vi "S4GUI_002.vi"(7 "Tab ObsEng":enum32{"Obs", "CCD modes", "Eng"}(tab)) -> ()   [LabVIEW 2018] (continued)
            n3950 = call-dynamic "Read AcquisitionA.vi"("error in (no error)"=w9244, "S4ACS_GUI in"=w9246) -> ("error out"=w9249:errorcluster, "Acquisition.lvclass"=w9248:refnum<class "Acquisition.lvclass">, "S4ACS_GUI out"=w9245:refnum<class "S4GUI.lvclass">)  [unwired: 7 in]
            n3951 = call-dynamic "Read Channel.vi"("error in (no error)"=w9249, "Acquisition in"=w9248) -> ("error out"=w9251:errorcluster, "Channel.lvclass"=w9250:refnum<class "Channel.lvclass">, "Acquisition out"=w9259:refnum<class "Acquisition.lvclass">)  [unwired: 7 in]
            n3952 = call-dynamic "Read State Machine.vi"("error in (no error)"=w9251, "Device in"=w9250) -> ("error out"=w9253:errorcluster, "State Machine.lvclass"=w9252:refnum<class "State Machine.lvclass">, "Device out"=w9255:refnum<class "Channel.lvclass">)  [unwired: 7 in]
            n3953 = call "Next State.vi"("error in (no error)"=w9253, "New_State"=u32 80, "State Machine in"=w9252) -> ("error out"=w9256:errorcluster, "State Machine out"=w9254:refnum<class "State Machine.lvclass">)  [unwired: 7 in]
            n3954 = call-dynamic "Write State Machine.vi"("error in (no error)"=w9256, "State Machine.lvclass"=w9254, "Device in"=w9255) -> ("error out"=w9260:errorcluster, "Device out"=w9261:refnum<class "Channel.lvclass">)  [unwired: 7 in]
            n3955 = call-dynamic "Write Channel.vi"("error in (no error)"=w9260, "Channel.lvclass"=w9261, "Acquisition in"=w9259) -> ("error out"=w9258:errorcluster, "Acquisition out"=w9257:refnum<class "Acquisition.lvclass">)  [unwired: 7 in]
            n3956 = call-dynamic "Write AcquisitionA.vi"("error in (no error)"=w9258, "Acquisition.lvclass"=w9257, "S4ACS_GUI in"=w9245) -> ("error out"=w9230:errorcluster, "S4ACS_GUI out"=w9229:refnum<class "S4GUI.lvclass">)  [unwired: 7 in]
            n3957 = call "Read AcquisitionB.vi"("error in (no error)"=w9230, "S4ACS_GUI in"=w9229) -> ("error out"=w9223:errorcluster, "Acquisition.lvclass"=w9227:refnum<class "Acquisition.lvclass">, "S4ACS_GUI out"=w9228:refnum<class "S4GUI.lvclass">)  [unwired: 7 in]
            n3958 = call-dynamic "Read Channel.vi"("error in (no error)"=w9223, "Acquisition in"=w9227) -> ("error out"=w9238:errorcluster, "Channel.lvclass"=w9239:refnum<class "Channel.lvclass">, "Acquisition out"=w9225:refnum<class "Acquisition.lvclass">)  [unwired: 7 in]
            n3959 = call-dynamic "Read State Machine.vi"("error in (no error)"=w9238, "Device in"=w9239) -> ("error out"=w9236:errorcluster, "State Machine.lvclass"=w9237:refnum<class "State Machine.lvclass">, "Device out"=w9234:refnum<class "Channel.lvclass">)  [unwired: 7 in]
            n3960 = call "Next State.vi"("error in (no error)"=w9236, "New_State"=u32 80, "State Machine in"=w9237) -> ("error out"=w9233:errorcluster, "State Machine out"=w9235:refnum<class "State Machine.lvclass">)  [unwired: 7 in]
            n3961 = call-dynamic "Write State Machine.vi"("error in (no error)"=w9233, "State Machine.lvclass"=w9235, "Device in"=w9234) -> ("error out"=w9232:errorcluster, "Device out"=w9231:refnum<class "Channel.lvclass">)  [unwired: 7 in]
            n3962 = call-dynamic "Write Channel.vi"("error in (no error)"=w9232, "Channel.lvclass"=w9231, "Acquisition in"=w9225) -> ("error out"=w9224:errorcluster, "Acquisition out"=w9226:refnum<class "Acquisition.lvclass">)  [unwired: 7 in]
            n3963 = call "Write AcquisitionB.vi"("error in (no error)"=w9224, "Acquisition.lvclass"=w9226, "S4ACS_GUI in"=w9228) -> ("error out"=w9190:errorcluster, "S4ACS_GUI out"=w9189:refnum<class "S4GUI.lvclass">)  [unwired: 7 in]
            n3964 = call-dynamic "Read AcquisitionC.vi"("error in (no error)"=w9190, "S4ACS_GUI in"=w9189) -> ("error out"=w9207:errorcluster, "Acquisition.lvclass"=w9211:refnum<class "Acquisition.lvclass">, "S4ACS_GUI out"=w9212:refnum<class "S4GUI.lvclass">)  [unwired: 7 in]
            n3965 = call-dynamic "Read Channel.vi"("error in (no error)"=w9207, "Acquisition in"=w9211) -> ("error out"=w9220:errorcluster, "Channel.lvclass"=w9221:refnum<class "Channel.lvclass">, "Acquisition out"=w9209:refnum<class "Acquisition.lvclass">)  [unwired: 7 in]
            n3966 = call-dynamic "Read State Machine.vi"("error in (no error)"=w9220, "Device in"=w9221) -> ("error out"=w9218:errorcluster, "State Machine.lvclass"=w9219:refnum<class "State Machine.lvclass">, "Device out"=w9216:refnum<class "Channel.lvclass">)  [unwired: 7 in]
            n3967 = call "Next State.vi"("error in (no error)"=w9218, "New_State"=u32 80, "State Machine in"=w9219) -> ("error out"=w9215:errorcluster, "State Machine out"=w9217:refnum<class "State Machine.lvclass">)  [unwired: 7 in]
            n3968 = call-dynamic "Write State Machine.vi"("error in (no error)"=w9215, "State Machine.lvclass"=w9217, "Device in"=w9216) -> ("error out"=w9214:errorcluster, "Device out"=w9213:refnum<class "Channel.lvclass">)  [unwired: 7 in]
            n3969 = call-dynamic "Write Channel.vi"("error in (no error)"=w9214, "Channel.lvclass"=w9213, "Acquisition in"=w9209) -> ("error out"=w9208:errorcluster, "Acquisition out"=w9210:refnum<class "Acquisition.lvclass">)  [unwired: 7 in]
            n3970 = call-dynamic "Write AcquisitionC.vi"("error in (no error)"=w9208, "Acquisition.lvclass"=w9210, "S4ACS_GUI in"=w9212) -> ("error out"=w9188:errorcluster, "S4ACS_GUI out"=w9187:refnum<class "S4GUI.lvclass">)  [unwired: 7 in]
            n3971 = call-dynamic "Read AcquisitionD.vi"("error in (no error)"=w9188, "S4ACS_GUI in"=w9187) -> ("error out"=w9191:errorcluster, "Acquisition.lvclass"=w9195:refnum<class "Acquisition.lvclass">, "S4ACS_GUI out"=w9196:refnum<class "S4GUI.lvclass">)  [unwired: 7 in]
            n3972 = call-dynamic "Read Channel.vi"("error in (no error)"=w9191, "Acquisition in"=w9195) -> ("error out"=w9204:errorcluster, "Channel.lvclass"=w9205:refnum<class "Channel.lvclass">, "Acquisition out"=w9193:refnum<class "Acquisition.lvclass">)  [unwired: 7 in]
            n3973 = call-dynamic "Read State Machine.vi"("error in (no error)"=w9204, "Device in"=w9205) -> ("error out"=w9202:errorcluster, "State Machine.lvclass"=w9203:refnum<class "State Machine.lvclass">, "Device out"=w9200:refnum<class "Channel.lvclass">)  [unwired: 7 in]
            n3974 = call "Next State.vi"("error in (no error)"=w9202, "New_State"=u32 80, "State Machine in"=w9203) -> ("error out"=w9199:errorcluster, "State Machine out"=w9201:refnum<class "State Machine.lvclass">)  [unwired: 7 in]
            n3975 = call-dynamic "Write State Machine.vi"("error in (no error)"=w9199, "State Machine.lvclass"=w9201, "Device in"=w9200) -> ("error out"=w9198:errorcluster, "Device out"=w9197:refnum<class "Channel.lvclass">)  [unwired: 7 in]
            n3976 = call-dynamic "Write Channel.vi"("error in (no error)"=w9198, "Channel.lvclass"=w9197, "Acquisition in"=w9193) -> ("error out"=w9192:errorcluster, "Acquisition out"=w9194:refnum<class "Acquisition.lvclass">)  [unwired: 7 in]
            n3977 = call-dynamic "Write AcquisitionD.vi"("error in (no error)"=w9192, "Acquisition.lvclass"=w9194, "S4ACS_GUI in"=w9196) -> ("error out"=w9185:errorcluster, "S4ACS_GUI out"=w9186:refnum<class "S4GUI.lvclass">)  [unwired: 7 in]
            n3978 = disable-structure shown="Enabled" {
              disable-tunnel: w9186 -> [w9266 w9268]
              disable-tunnel: w9185 -> [w9265 w9267]
              disable-tunnel: [w9263 w9268] -> w9242
              disable-tunnel: [w9262 w9267] -> w9241
              frame Disabled {
                n3979 = call-dynamic "Write aborted.vi"("error in (no error)"=w9265, "aborted"=TRUE ("stopped"), "S4ACS_GUI in"=w9266) -> ("error out"=w9262:errorcluster, "S4ACS_GUI out"=w9263:refnum<class "S4GUI.lvclass">)  [unwired: 7 in]
              }
              frame Enabled {
              }
            }
            n3980 = call-dynamic "Write Obs_state.vi"("error in (no error)"=w9241, "Obs_state"=u32 0, "S4ACS_GUI in"=w9242) -> ("error out"=w9159:errorcluster, "S4ACS_GUI out"=w9160:refnum<class "S4GUI.lvclass">)  [unwired: 7 in]
            n3981 = call "Read Instrument.lvclass.vi"("error in (no error)"=w9159, "S4ACS_GUI in"=w9160) -> ("error out"=w9179:errorcluster, "Instrument.lvclass"=w9181:refnum<class "Instrument.lvclass">, "S4ACS_GUI out"=w9180:refnum<class "S4GUI.lvclass">)  [unwired: 7 in]
            n3982 = call "Read WPROT.vi"("error in (no error)"=w9179, "Instrument in"=w9181) -> ("error out"=w9174:errorcluster, "Opt_Selector.lvclass"=w9177:refnum<class "Opt_Selector.lvclass">, "Instrument out"=w9182:refnum<class "Instrument.lvclass">)  [unwired: 7 in]
            n3983 = call-dynamic "Read sequencia_ant.vi"("error in (no error)"=w9174, "Opt_Selector in"=w9177) -> ("error out"=w9173:errorcluster, "sequencia_ant"=w9175:u16, "Opt_Selector out"=w9176:refnum<class "Opt_Selector.lvclass">)  [unwired: 7 in]
            n3984 = call-dynamic "Write sequencia.vi"("error in (no error)"=w9173, "sequencia"=w9175, "Opt_Selector in"=w9176) -> ("error out"=w9168:errorcluster, "Opt_Selector out"=w9169:refnum<class "Opt_Selector.lvclass">)  [unwired: 7 in]
            n3985 = call-dynamic "Read State Machine.vi"("error in (no error)"=w9168, "Device in"=w9169) -> ("error out"=w9171:errorcluster, "State Machine.lvclass"=w9166:refnum<class "State Machine.lvclass">, "Device out"=w9167:refnum<class "Opt_Selector.lvclass">)  [unwired: 7 in]
            n3986 = call "Next State.vi"("error in (no error)"=w9171, "New_State"=10, "State Machine in"=w9166) -> ("error out"=w9170:errorcluster, "State Machine out"=w9165:refnum<class "State Machine.lvclass">)  [unwired: 7 in]
            n3987 = call-dynamic "Write State Machine.vi"("error in (no error)"=w9170, "State Machine.lvclass"=w9165, "Device in"=w9167) -> ("error out"=w9164:errorcluster, "Device out"=w9163:refnum<class "Opt_Selector.lvclass">)  [unwired: 7 in]
            n3988 = call "Write WPROT.vi"("error in (no error)"=w9164, "Opt_Selector.lvclass"=w9163, "Instrument in"=w9182) -> ("error out"=w9161:errorcluster, "Instrument out"=w9162:refnum<class "Instrument.lvclass">)  [unwired: 7 in]
            n3989 = call "Write Instrument.lvclass.vi"("error in (no error)"=w9161, "Instrument.lvclass"=w9162, "S4ACS_GUI in"=w9180) -> ("error out"=w9183:errorcluster, "S4ACS_GUI out"=w9184:refnum<class "S4GUI.lvclass">)  [unwired: 7 in]
            n3990 = call-dynamic "Write ciclos.vi"("error in (no error)"=w9183, "ciclos"=u32 0, "S4ACS_GUI in"=w9184) -> ("error out"=w9157:errorcluster, "S4ACS_GUI out"=w9158:refnum<class "S4GUI.lvclass">)  [unwired: 7 in]
          }
          frame Enabled {
            w9274 = FALSE ("Wait Until Done")
            n3991 = call <vilib>:"Application Directory.vi"() -> ("Application Directory"=w9269:path)
            n3992 = Build Path(base path=w9269, name or relative path="MsgAbortSync.vi") -> (appended path=w9277:path)
            n3993 = Open VI Reference(vi path=w9277, error in (no error)=w9272) -> (vi reference=w9276:refnum<vi>, error out=w9275:errorcluster)  [unwired: 4 in]
            n3994 = invoke class="VI" method="Run VI"(reference=w9276, error in=w9275, "Wait until done"=w9274, "Auto Dispose Ref"=w9274) -> (error out=w9271:errorcluster)  [unwired: 1 in, 4 out]
          }
        }
        n3995 = property on="#Cycles Done" class="Slide (strict)"(error in=w9153, "Scale.Maximum"=w9155, "Scale.Minimum"=w9155) -> (error out=w9156:errorcluster)  [unwired: 1 in, 1 out]
      }
      event "Pause SM": Value Change {
        n3996 = event-data() -> ()  [unwired: 1 in, 6 out]
        n3997 = call-dynamic "Write User Event.vi"("error in (no error)"=w9281, "User Event"="PAUSE SM CLICKED", "S4GUI in"=w9282) -> ("error out"=w9279:errorcluster, "S4GUI out"=w9280:refnum<class "S4GUI.lvclass">)  [unwired: 7 in]
        n3998 = disable-structure shown="Enabled" {
          disable-tunnel: w9280 -> [w9296 w9306]
          disable-tunnel: w9279 -> [w9295 w9307]
          disable-tunnel: [w9286 w9306] -> w9284
          disable-tunnel: [w9285 w9305] -> w9283
          frame Disabled {
            n3999 = disable-structure shown="Enabled" {
              disable-tunnel: w9296 -> [w9300 w9303]
              disable-tunnel: w9295 -> [w9299 w9302]
              disable-tunnel: [w9298 w9303] -> w9289
              disable-tunnel: [w9297 w9302] -> w9288
              frame Disabled {
                n4000 = call-dynamic "Write paused.vi"("error in (no error)"=w9299, "paused"=TRUE ("stopped"), "S4ACS_GUI in"=w9300) -> ("error out"=w9297:errorcluster, "S4ACS_GUI out"=w9298:refnum<class "S4GUI.lvclass">)  [unwired: 7 in]
              }
              frame Enabled {
              }
            }
            n4001 = call-dynamic "Read Obs_state.vi"("error in (no error)"=w9288, "S4ACS_GUI in"=w9289) -> ("error out"=w9292:errorcluster, "Obs_state"=w9294:u32, "S4ACS_GUI out"=w9293:refnum<class "S4GUI.lvclass">)  [unwired: 7 in]
            n4002 = call-dynamic "Write Obs_prevstate.vi"("error in (no error)"=w9292, "Obs_prevstate"=w9294, "S4ACS_GUI in"=w9293) -> ("error out"=w9290:errorcluster, "S4ACS_GUI out"=w9291:refnum<class "S4GUI.lvclass">)  [unwired: 7 in]
            n4003 = call-dynamic "Write Obs_state.vi"("error in (no error)"=w9290, "Obs_state"=u32 400, "S4ACS_GUI in"=w9291) -> ("error out"=w9285:errorcluster, "S4ACS_GUI out"=w9286:refnum<class "S4GUI.lvclass">)  [unwired: 7 in]
          }
          frame Enabled {
            w9309 = FALSE ("Wait Until Done")
            n4004 = call <vilib>:"Application Directory.vi"() -> ("Application Directory"=w9304:path)
            n4005 = Build Path(base path=w9304, name or relative path="MsgPauseSync.vi") -> (appended path=w9312:path)
            n4006 = Open VI Reference(vi path=w9312, error in (no error)=w9307) -> (vi reference=w9311:refnum<vi>, error out=w9310:errorcluster)  [unwired: 4 in]
            n4007 = invoke class="VI" method="Run VI"(reference=w9311, error in=w9310, "Wait until done"=w9309, "Auto Dispose Ref"=w9309) -> (error out=w9305:errorcluster)  [unwired: 1 in, 4 out]
          }
        }
      }
      event "Abort ch1": Value Change {
        n4008 = event-data() -> ()  [unwired: 1 in, 6 out]
        n4009 = disable-structure shown="Enabled" {
          disable-tunnel: w9316 -> [w9349 w9371]
          disable-tunnel: w9315 -> [w9347 w9365]
          disable-tunnel: [w9329 w9364] -> w9314
          disable-tunnel: [w9317 w9371] -> w9313
          frame Disabled {
            # "Para movimento \nda lamina retardadora"
            # "Restaura a última sequência de lâminas"
            n4010 = call-dynamic "Read AcquisitionA.vi"("error in (no error)"=w9347, "S4ACS_GUI in"=w9349) -> ("error out"=w9352:errorcluster, "Acquisition.lvclass"=w9351:refnum<class "Acquisition.lvclass">, "S4ACS_GUI out"=w9348:refnum<class "S4GUI.lvclass">)  [unwired: 7 in]
            n4011 = call-dynamic "Read Channel.vi"("error in (no error)"=w9352, "Acquisition in"=w9351) -> ("error out"=w9354:errorcluster, "Channel.lvclass"=w9353:refnum<class "Channel.lvclass">, "Acquisition out"=w9360:refnum<class "Acquisition.lvclass">)  [unwired: 7 in]
            n4012 = call-dynamic "Read State Machine.vi"("error in (no error)"=w9354, "Device in"=w9353) -> ("error out"=w9356:errorcluster, "State Machine.lvclass"=w9355:refnum<class "State Machine.lvclass">, "Device out"=w9358:refnum<class "Channel.lvclass">)  [unwired: 7 in]
            n4013 = call "Next State.vi"("error in (no error)"=w9356, "New_State"=u32 80, "State Machine in"=w9355) -> ("error out"=w9359:errorcluster, "State Machine out"=w9357:refnum<class "State Machine.lvclass">)  [unwired: 7 in]
            n4014 = call-dynamic "Write State Machine.vi"("error in (no error)"=w9359, "State Machine.lvclass"=w9357, "Device in"=w9358) -> ("error out"=w9361:errorcluster, "Device out"=w9362:refnum<class "Channel.lvclass">)  [unwired: 7 in]
            n4015 = call-dynamic "Write Channel.vi"("error in (no error)"=w9361, "Channel.lvclass"=w9362, "Acquisition in"=w9360) -> ("error out"=w9344:errorcluster, "Acquisition out"=w9345:refnum<class "Acquisition.lvclass">)  [unwired: 7 in]
            n4016 = call-dynamic "Write Acq_state.vi"("error in (no error)"=w9344, "Acq_state"=u32 0, "Acquisition in"=w9345) -> ("error out"=w9343:errorcluster, "Acquisition out"=w9342:refnum<class "Acquisition.lvclass">)  [unwired: 7 in]
            n4017 = call-dynamic "Write AcquisitionA.vi"("error in (no error)"=w9343, "Acquisition.lvclass"=w9342, "S4ACS_GUI in"=w9348) -> ("error out"=w9330:errorcluster, "S4ACS_GUI out"=w9328:refnum<class "S4GUI.lvclass">)  [unwired: 7 in]
            n4018 = call "Read Instrument.lvclass.vi"("error in (no error)"=w9330, "S4ACS_GUI in"=w9328) -> ("error out"=w9337:errorcluster, "Instrument.lvclass"=w9340:refnum<class "Instrument.lvclass">, "S4ACS_GUI out"=w9341:refnum<class "S4GUI.lvclass">)  [unwired: 7 in]
            n4019 = call "Read WPROT.vi"("error in (no error)"=w9337, "Instrument in"=w9340) -> ("error out"=w9336:errorcluster, "Opt_Selector.lvclass"=w9338:refnum<class "Opt_Selector.lvclass">, "Instrument out"=w9339:refnum<class "Instrument.lvclass">)  [unwired: 7 in]
            n4020 = call-dynamic "Read sequencia_ant.vi"("error in (no error)"=w9336, "Opt_Selector in"=w9338) -> ("error out"=w9332:errorcluster, "sequencia_ant"=w9331:u16, "Opt_Selector out"=w9333:refnum<class "Opt_Selector.lvclass">)  [unwired: 7 in]
            n4021 = call-dynamic "Write sequencia.vi"("error in (no error)"=w9332, "sequencia"=w9331, "Opt_Selector in"=w9333) -> ("error out"=w9321:errorcluster, "Opt_Selector out"=w9322:refnum<class "Opt_Selector.lvclass">)  [unwired: 7 in]
            n4022 = call-dynamic "Read State Machine.vi"("error in (no error)"=w9321, "Device in"=w9322) -> ("error out"=w9324:errorcluster, "State Machine.lvclass"=w9327:refnum<class "State Machine.lvclass">, "Device out"=w9320:refnum<class "Opt_Selector.lvclass">)  [unwired: 7 in]
            n4023 = call "Next State.vi"("error in (no error)"=w9324, "New_State"=10, "State Machine in"=w9327) -> ("error out"=w9323:errorcluster, "State Machine out"=w9326:refnum<class "State Machine.lvclass">)  [unwired: 7 in]
            n4024 = call-dynamic "Write State Machine.vi"("error in (no error)"=w9323, "State Machine.lvclass"=w9326, "Device in"=w9320) -> ("error out"=w9318:errorcluster, "Device out"=w9319:refnum<class "Opt_Selector.lvclass">)  [unwired: 7 in]
            n4025 = call "Write WPROT.vi"("error in (no error)"=w9318, "Opt_Selector.lvclass"=w9319, "Instrument in"=w9339) -> ("error out"=w9335:errorcluster, "Instrument out"=w9334:refnum<class "Instrument.lvclass">)  [unwired: 7 in]
            n4026 = call "Write Instrument.lvclass.vi"("error in (no error)"=w9335, "Instrument.lvclass"=w9334, "S4ACS_GUI in"=w9341) -> ("error out"=w9329:errorcluster, "S4ACS_GUI out"=w9317:refnum<class "S4GUI.lvclass">)  [unwired: 7 in]
          }
          frame Enabled {
            w9367 = FALSE ("Wait Until Done")
            n4027 = call <vilib>:"Application Directory.vi"() -> ("Application Directory"=w9363:path)
            n4028 = Build Path(base path=w9363, name or relative path="MsgAbort1.vi") -> (appended path=w9370:path)
            n4029 = Open VI Reference(vi path=w9370, error in (no error)=w9365) -> (vi reference=w9369:refnum<vi>, error out=w9368:errorcluster)  [unwired: 4 in]
            n4030 = invoke class="VI" method="Run VI"(reference=w9369, error in=w9368, "Wait until done"=w9367, "Auto Dispose Ref"=w9367) -> (error out=w9364:errorcluster)  [unwired: 1 in, 4 out]
          }
        }
      }
      event "Abort ch2": Value Change {
        n4031 = event-data() -> ()  [unwired: 1 in, 6 out]
        n4032 = disable-structure shown="Enabled" {
          disable-tunnel: w9375 -> [w9408 w9424]
          disable-tunnel: w9374 -> [w9406 w9425]
          disable-tunnel: [w9388 w9423] -> w9373
          disable-tunnel: [w9376 w9424] -> w9372
          frame Disabled {
            # "Para movimento \nda lamina retardadora"
            # "Restaura a última sequência de lâminas"
            n4033 = call "Read AcquisitionB.vi"("error in (no error)"=w9406, "S4ACS_GUI in"=w9408) -> ("error out"=w9411:errorcluster, "Acquisition.lvclass"=w9410:refnum<class "Acquisition.lvclass">, "S4ACS_GUI out"=w9407:refnum<class "S4GUI.lvclass">)  [unwired: 7 in]
            n4034 = call-dynamic "Read Channel.vi"("error in (no error)"=w9411, "Acquisition in"=w9410) -> ("error out"=w9413:errorcluster, "Channel.lvclass"=w9412:refnum<class "Channel.lvclass">, "Acquisition out"=w9419:refnum<class "Acquisition.lvclass">)  [unwired: 7 in]
            n4035 = call-dynamic "Read State Machine.vi"("error in (no error)"=w9413, "Device in"=w9412) -> ("error out"=w9415:errorcluster, "State Machine.lvclass"=w9414:refnum<class "State Machine.lvclass">, "Device out"=w9417:refnum<class "Channel.lvclass">)  [unwired: 7 in]
            n4036 = call "Next State.vi"("error in (no error)"=w9415, "New_State"=u32 80, "State Machine in"=w9414) -> ("error out"=w9418:errorcluster, "State Machine out"=w9416:refnum<class "State Machine.lvclass">)  [unwired: 7 in]
            n4037 = call-dynamic "Write State Machine.vi"("error in (no error)"=w9418, "State Machine.lvclass"=w9416, "Device in"=w9417) -> ("error out"=w9420:errorcluster, "Device out"=w9421:refnum<class "Channel.lvclass">)  [unwired: 7 in]
            n4038 = call-dynamic "Write Channel.vi"("error in (no error)"=w9420, "Channel.lvclass"=w9421, "Acquisition in"=w9419) -> ("error out"=w9403:errorcluster, "Acquisition out"=w9404:refnum<class "Acquisition.lvclass">)  [unwired: 7 in]
            n4039 = call-dynamic "Write Acq_state.vi"("error in (no error)"=w9403, "Acq_state"=u32 0, "Acquisition in"=w9404) -> ("error out"=w9402:errorcluster, "Acquisition out"=w9401:refnum<class "Acquisition.lvclass">)  [unwired: 7 in]
            n4040 = call "Write AcquisitionB.vi"("error in (no error)"=w9402, "Acquisition.lvclass"=w9401, "S4ACS_GUI in"=w9407) -> ("error out"=w9389:errorcluster, "S4ACS_GUI out"=w9387:refnum<class "S4GUI.lvclass">)  [unwired: 7 in]
            n4041 = call "Read Instrument.lvclass.vi"("error in (no error)"=w9389, "S4ACS_GUI in"=w9387) -> ("error out"=w9396:errorcluster, "Instrument.lvclass"=w9399:refnum<class "Instrument.lvclass">, "S4ACS_GUI out"=w9400:refnum<class "S4GUI.lvclass">)  [unwired: 7 in]
            n4042 = call "Read WPROT.vi"("error in (no error)"=w9396, "Instrument in"=w9399) -> ("error out"=w9395:errorcluster, "Opt_Selector.lvclass"=w9397:refnum<class "Opt_Selector.lvclass">, "Instrument out"=w9398:refnum<class "Instrument.lvclass">)  [unwired: 7 in]
            n4043 = call-dynamic "Read sequencia_ant.vi"("error in (no error)"=w9395, "Opt_Selector in"=w9397) -> ("error out"=w9391:errorcluster, "sequencia_ant"=w9390:u16, "Opt_Selector out"=w9392:refnum<class "Opt_Selector.lvclass">)  [unwired: 7 in]
            n4044 = call-dynamic "Write sequencia.vi"("error in (no error)"=w9391, "sequencia"=w9390, "Opt_Selector in"=w9392) -> ("error out"=w9380:errorcluster, "Opt_Selector out"=w9381:refnum<class "Opt_Selector.lvclass">)  [unwired: 7 in]
            n4045 = call-dynamic "Read State Machine.vi"("error in (no error)"=w9380, "Device in"=w9381) -> ("error out"=w9383:errorcluster, "State Machine.lvclass"=w9386:refnum<class "State Machine.lvclass">, "Device out"=w9379:refnum<class "Opt_Selector.lvclass">)  [unwired: 7 in]
            n4046 = call "Next State.vi"("error in (no error)"=w9383, "New_State"=10, "State Machine in"=w9386) -> ("error out"=w9382:errorcluster, "State Machine out"=w9385:refnum<class "State Machine.lvclass">)  [unwired: 7 in]
            n4047 = call-dynamic "Write State Machine.vi"("error in (no error)"=w9382, "State Machine.lvclass"=w9385, "Device in"=w9379) -> ("error out"=w9377:errorcluster, "Device out"=w9378:refnum<class "Opt_Selector.lvclass">)  [unwired: 7 in]
            n4048 = call "Write WPROT.vi"("error in (no error)"=w9377, "Opt_Selector.lvclass"=w9378, "Instrument in"=w9398) -> ("error out"=w9394:errorcluster, "Instrument out"=w9393:refnum<class "Instrument.lvclass">)  [unwired: 7 in]
            n4049 = call "Write Instrument.lvclass.vi"("error in (no error)"=w9394, "Instrument.lvclass"=w9393, "S4ACS_GUI in"=w9400) -> ("error out"=w9388:errorcluster, "S4ACS_GUI out"=w9376:refnum<class "S4GUI.lvclass">)  [unwired: 7 in]
          }
          frame Enabled {
            w9427 = FALSE ("Wait Until Done")
            n4050 = call <vilib>:"Application Directory.vi"() -> ("Application Directory"=w9422:path)
            n4051 = Build Path(base path=w9422, name or relative path="MsgAbort2.vi") -> (appended path=w9430:path)
            n4052 = Open VI Reference(vi path=w9430, error in (no error)=w9425) -> (vi reference=w9429:refnum<vi>, error out=w9428:errorcluster)  [unwired: 4 in]
            n4053 = invoke class="VI" method="Run VI"(reference=w9429, error in=w9428, "Wait until done"=w9427, "Auto Dispose Ref"=w9427) -> (error out=w9423:errorcluster)  [unwired: 1 in, 4 out]
          }
        }
      }
      event "Abort ch3": Value Change {
        n4054 = event-data() -> ()  [unwired: 1 in, 6 out]
        n4055 = disable-structure shown="Enabled" {
          disable-tunnel: w9434 -> [w9467 w9483]
          disable-tunnel: w9433 -> [w9465 w9484]
          disable-tunnel: [w9447 w9482] -> w9432
          disable-tunnel: [w9435 w9483] -> w9431
          frame Disabled {
            # "Para movimento \nda lamina retardadora"
            # "Restaura a última sequência de lâminas"
            n4056 = call-dynamic "Read AcquisitionC.vi"("error in (no error)"=w9465, "S4ACS_GUI in"=w9467) -> ("error out"=w9470:errorcluster, "Acquisition.lvclass"=w9469:refnum<class "Acquisition.lvclass">, "S4ACS_GUI out"=w9466:refnum<class "S4GUI.lvclass">)  [unwired: 7 in]
            n4057 = call-dynamic "Read Channel.vi"("error in (no error)"=w9470, "Acquisition in"=w9469) -> ("error out"=w9472:errorcluster, "Channel.lvclass"=w9471:refnum<class "Channel.lvclass">, "Acquisition out"=w9478:refnum<class "Acquisition.lvclass">)  [unwired: 7 in]
            n4058 = call-dynamic "Read State Machine.vi"("error in (no error)"=w9472, "Device in"=w9471) -> ("error out"=w9474:errorcluster, "State Machine.lvclass"=w9473:refnum<class "State Machine.lvclass">, "Device out"=w9476:refnum<class "Channel.lvclass">)  [unwired: 7 in]
            n4059 = call "Next State.vi"("error in (no error)"=w9474, "New_State"=u32 80, "State Machine in"=w9473) -> ("error out"=w9477:errorcluster, "State Machine out"=w9475:refnum<class "State Machine.lvclass">)  [unwired: 7 in]
            n4060 = call-dynamic "Write State Machine.vi"("error in (no error)"=w9477, "State Machine.lvclass"=w9475, "Device in"=w9476) -> ("error out"=w9479:errorcluster, "Device out"=w9480:refnum<class "Channel.lvclass">)  [unwired: 7 in]
            n4061 = call-dynamic "Write Channel.vi"("error in (no error)"=w9479, "Channel.lvclass"=w9480, "Acquisition in"=w9478) -> ("error out"=w9462:errorcluster, "Acquisition out"=w9463:refnum<class "Acquisition.lvclass">)  [unwired: 7 in]
            n4062 = call-dynamic "Write Acq_state.vi"("error in (no error)"=w9462, "Acq_state"=u32 0, "Acquisition in"=w9463) -> ("error out"=w9461:errorcluster, "Acquisition out"=w9460:refnum<class "Acquisition.lvclass">)  [unwired: 7 in]
            n4063 = call-dynamic "Write AcquisitionC.vi"("error in (no error)"=w9461, "Acquisition.lvclass"=w9460, "S4ACS_GUI in"=w9466) -> ("error out"=w9448:errorcluster, "S4ACS_GUI out"=w9446:refnum<class "S4GUI.lvclass">)  [unwired: 7 in]
            n4064 = call "Read Instrument.lvclass.vi"("error in (no error)"=w9448, "S4ACS_GUI in"=w9446) -> ("error out"=w9455:errorcluster, "Instrument.lvclass"=w9458:refnum<class "Instrument.lvclass">, "S4ACS_GUI out"=w9459:refnum<class "S4GUI.lvclass">)  [unwired: 7 in]
            n4065 = call "Read WPROT.vi"("error in (no error)"=w9455, "Instrument in"=w9458) -> ("error out"=w9454:errorcluster, "Opt_Selector.lvclass"=w9456:refnum<class "Opt_Selector.lvclass">, "Instrument out"=w9457:refnum<class "Instrument.lvclass">)  [unwired: 7 in]
            n4066 = call-dynamic "Read sequencia_ant.vi"("error in (no error)"=w9454, "Opt_Selector in"=w9456) -> ("error out"=w9450:errorcluster, "sequencia_ant"=w9449:u16, "Opt_Selector out"=w9451:refnum<class "Opt_Selector.lvclass">)  [unwired: 7 in]
            n4067 = call-dynamic "Write sequencia.vi"("error in (no error)"=w9450, "sequencia"=w9449, "Opt_Selector in"=w9451) -> ("error out"=w9439:errorcluster, "Opt_Selector out"=w9440:refnum<class "Opt_Selector.lvclass">)  [unwired: 7 in]
            n4068 = call-dynamic "Read State Machine.vi"("error in (no error)"=w9439, "Device in"=w9440) -> ("error out"=w9442:errorcluster, "State Machine.lvclass"=w9445:refnum<class "State Machine.lvclass">, "Device out"=w9438:refnum<class "Opt_Selector.lvclass">)  [unwired: 7 in]
            n4069 = call "Next State.vi"("error in (no error)"=w9442, "New_State"=10, "State Machine in"=w9445) -> ("error out"=w9441:errorcluster, "State Machine out"=w9444:refnum<class "State Machine.lvclass">)  [unwired: 7 in]
            n4070 = call-dynamic "Write State Machine.vi"("error in (no error)"=w9441, "State Machine.lvclass"=w9444, "Device in"=w9438) -> ("error out"=w9436:errorcluster, "Device out"=w9437:refnum<class "Opt_Selector.lvclass">)  [unwired: 7 in]
            n4071 = call "Write WPROT.vi"("error in (no error)"=w9436, "Opt_Selector.lvclass"=w9437, "Instrument in"=w9457) -> ("error out"=w9453:errorcluster, "Instrument out"=w9452:refnum<class "Instrument.lvclass">)  [unwired: 7 in]
            n4072 = call "Write Instrument.lvclass.vi"("error in (no error)"=w9453, "Instrument.lvclass"=w9452, "S4ACS_GUI in"=w9459) -> ("error out"=w9447:errorcluster, "S4ACS_GUI out"=w9435:refnum<class "S4GUI.lvclass">)  [unwired: 7 in]
          }
          frame Enabled {
            w9486 = FALSE ("Wait Until Done")
            n4073 = call <vilib>:"Application Directory.vi"() -> ("Application Directory"=w9481:path)
            n4074 = Build Path(base path=w9481, name or relative path="MsgAbort3.vi") -> (appended path=w9489:path)
            n4075 = Open VI Reference(vi path=w9489, error in (no error)=w9484) -> (vi reference=w9488:refnum<vi>, error out=w9487:errorcluster)  [unwired: 4 in]
            n4076 = invoke class="VI" method="Run VI"(reference=w9488, error in=w9487, "Wait until done"=w9486, "Auto Dispose Ref"=w9486) -> (error out=w9482:errorcluster)  [unwired: 1 in, 4 out]
          }
        }
      }
      event "Abort ch4": Value Change {
        n4077 = event-data() -> ()  [unwired: 1 in, 6 out]
        n4078 = disable-structure shown="Enabled" {
          disable-tunnel: w9493 -> [w9526 w9542]
          disable-tunnel: w9492 -> [w9524 w9543]
          disable-tunnel: [w9506 w9541] -> w9491
          disable-tunnel: [w9494 w9542] -> w9490
          frame Disabled {
            # "Para movimento \nda lamina retardadora"
            # "Restaura a última sequência de lâminas"
            n4079 = call-dynamic "Read AcquisitionD.vi"("error in (no error)"=w9524, "S4ACS_GUI in"=w9526) -> ("error out"=w9529:errorcluster, "Acquisition.lvclass"=w9528:refnum<class "Acquisition.lvclass">, "S4ACS_GUI out"=w9525:refnum<class "S4GUI.lvclass">)  [unwired: 7 in]
            n4080 = call-dynamic "Read Channel.vi"("error in (no error)"=w9529, "Acquisition in"=w9528) -> ("error out"=w9531:errorcluster, "Channel.lvclass"=w9530:refnum<class "Channel.lvclass">, "Acquisition out"=w9537:refnum<class "Acquisition.lvclass">)  [unwired: 7 in]
            n4081 = call-dynamic "Read State Machine.vi"("error in (no error)"=w9531, "Device in"=w9530) -> ("error out"=w9533:errorcluster, "State Machine.lvclass"=w9532:refnum<class "State Machine.lvclass">, "Device out"=w9535:refnum<class "Channel.lvclass">)  [unwired: 7 in]
            n4082 = call "Next State.vi"("error in (no error)"=w9533, "New_State"=u32 80, "State Machine in"=w9532) -> ("error out"=w9536:errorcluster, "State Machine out"=w9534:refnum<class "State Machine.lvclass">)  [unwired: 7 in]
            n4083 = call-dynamic "Write State Machine.vi"("error in (no error)"=w9536, "State Machine.lvclass"=w9534, "Device in"=w9535) -> ("error out"=w9538:errorcluster, "Device out"=w9539:refnum<class "Channel.lvclass">)  [unwired: 7 in]
            n4084 = call-dynamic "Write Channel.vi"("error in (no error)"=w9538, "Channel.lvclass"=w9539, "Acquisition in"=w9537) -> ("error out"=w9521:errorcluster, "Acquisition out"=w9522:refnum<class "Acquisition.lvclass">)  [unwired: 7 in]
            n4085 = call-dynamic "Write Acq_state.vi"("error in (no error)"=w9521, "Acq_state"=u32 0, "Acquisition in"=w9522) -> ("error out"=w9520:errorcluster, "Acquisition out"=w9519:refnum<class "Acquisition.lvclass">)  [unwired: 7 in]
            n4086 = call-dynamic "Write AcquisitionD.vi"("error in (no error)"=w9520, "Acquisition.lvclass"=w9519, "S4ACS_GUI in"=w9525) -> ("error out"=w9507:errorcluster, "S4ACS_GUI out"=w9505:refnum<class "S4GUI.lvclass">)  [unwired: 7 in]
            n4087 = call "Read Instrument.lvclass.vi"("error in (no error)"=w9507, "S4ACS_GUI in"=w9505) -> ("error out"=w9514:errorcluster, "Instrument.lvclass"=w9517:refnum<class "Instrument.lvclass">, "S4ACS_GUI out"=w9518:refnum<class "S4GUI.lvclass">)  [unwired: 7 in]
            n4088 = call "Read WPROT.vi"("error in (no error)"=w9514, "Instrument in"=w9517) -> ("error out"=w9513:errorcluster, "Opt_Selector.lvclass"=w9515:refnum<class "Opt_Selector.lvclass">, "Instrument out"=w9516:refnum<class "Instrument.lvclass">)  [unwired: 7 in]
            n4089 = call-dynamic "Read sequencia_ant.vi"("error in (no error)"=w9513, "Opt_Selector in"=w9515) -> ("error out"=w9509:errorcluster, "sequencia_ant"=w9508:u16, "Opt_Selector out"=w9510:refnum<class "Opt_Selector.lvclass">)  [unwired: 7 in]
            n4090 = call-dynamic "Write sequencia.vi"("error in (no error)"=w9509, "sequencia"=w9508, "Opt_Selector in"=w9510) -> ("error out"=w9498:errorcluster, "Opt_Selector out"=w9499:refnum<class "Opt_Selector.lvclass">)  [unwired: 7 in]
            n4091 = call-dynamic "Read State Machine.vi"("error in (no error)"=w9498, "Device in"=w9499) -> ("error out"=w9501:errorcluster, "State Machine.lvclass"=w9504:refnum<class "State Machine.lvclass">, "Device out"=w9497:refnum<class "Opt_Selector.lvclass">)  [unwired: 7 in]
            n4092 = call "Next State.vi"("error in (no error)"=w9501, "New_State"=10, "State Machine in"=w9504) -> ("error out"=w9500:errorcluster, "State Machine out"=w9503:refnum<class "State Machine.lvclass">)  [unwired: 7 in]
            n4093 = call-dynamic "Write State Machine.vi"("error in (no error)"=w9500, "State Machine.lvclass"=w9503, "Device in"=w9497) -> ("error out"=w9495:errorcluster, "Device out"=w9496:refnum<class "Opt_Selector.lvclass">)  [unwired: 7 in]
            n4094 = call "Write WPROT.vi"("error in (no error)"=w9495, "Opt_Selector.lvclass"=w9496, "Instrument in"=w9516) -> ("error out"=w9512:errorcluster, "Instrument out"=w9511:refnum<class "Instrument.lvclass">)  [unwired: 7 in]
            n4095 = call "Write Instrument.lvclass.vi"("error in (no error)"=w9512, "Instrument.lvclass"=w9511, "S4ACS_GUI in"=w9518) -> ("error out"=w9506:errorcluster, "S4ACS_GUI out"=w9494:refnum<class "S4GUI.lvclass">)  [unwired: 7 in]
          }
          frame Enabled {
            w9545 = FALSE ("Wait Until Done")
            n4096 = call <vilib>:"Application Directory.vi"() -> ("Application Directory"=w9540:path)
            n4097 = Build Path(base path=w9540, name or relative path="MsgAbort4.vi") -> (appended path=w9548:path)
            n4098 = Open VI Reference(vi path=w9548, error in (no error)=w9543) -> (vi reference=w9547:refnum<vi>, error out=w9546:errorcluster)  [unwired: 4 in]
            n4099 = invoke class="VI" method="Run VI"(reference=w9547, error in=w9546, "Wait until done"=w9545, "Auto Dispose Ref"=w9545) -> (error out=w9541:errorcluster)  [unwired: 1 in, 4 out]
          }
        }
      }
      event "SyncBox": Value Change {
        n4100 = event-data() -> ()  [unwired: 1 in, 4 out]
        n4101 = call-dynamic "Read Sync Box.lvclass.vi"("error in (no error)"=w9551, "SPARC4_AC in"=w9552) -> ("error out"=w9567:errorcluster, "Sync Box.lvclass"=w9568:refnum<class "Sync Box.lvclass">, "SPARC4_AC out"=w9556:refnum<class "S4GUI.lvclass">)  [unwired: 7 in]
        n4102 = call-dynamic "Read Trigger.lvclass.vi"("error in (no error)"=w9567, "Sync Box in"=w9568) -> ("error out"=w9565:errorcluster, "Trigger.lvclass"=w9566:refnum<class "Trigger.lvclass">, "Sync Box out"=w9559:refnum<class "Sync Box.lvclass">)  [unwired: 7 in]
        n4103 = call-dynamic "Read State Machine.vi"("error in (no error)"=w9565, "Device in"=w9566) -> ("error out"=w9563:errorcluster, "State Machine.lvclass"=w9564:refnum<class "State Machine.lvclass">, "Device out"=w9560:refnum<class "Trigger.lvclass">)  [unwired: 7 in]
        n4104 = call "Next State.vi"("error in (no error)"=w9563, "New_State"=u32 1, "State Machine in"=w9564) -> ("error out"=w9558:errorcluster, "State Machine out"=w9561:refnum<class "State Machine.lvclass">)  [unwired: 7 in]
        n4105 = call-dynamic "Write State Machine.vi"("error in (no error)"=w9558, "State Machine.lvclass"=w9561, "Device in"=w9560) -> ("error out"=w9554:errorcluster, "Device out"=w9553:refnum<class "Trigger.lvclass">)  [unwired: 7 in]
        n4106 = call-dynamic "Write Trigger.lvclass.vi"("error in (no error)"=w9554, "Trigger.lvclass"=w9553, "Sync Box in"=w9559) -> ("error out"=w9555:errorcluster, "Sync Box out"=w9557:refnum<class "Sync Box.lvclass">)  [unwired: 7 in]
        n4107 = call-dynamic "Write Sync Box.lvclass.vi"("error in (no error)"=w9555, "Sync Box.lvclass"=w9557, "SPARC4_AC in"=w9556) -> ("error out"=w9550:errorcluster, "SPARC4_AC out"=w9549:refnum<class "S4GUI.lvclass">)  [unwired: 7 in]
      }
      event "Fire manual", "Fire": Value Change {
        n4108 = event-data() -> ()  [unwired: 1 in, 4 out]
        n4109 = call-dynamic "Read Sync Box.lvclass.vi"("error in (no error)"=w9571, "SPARC4_AC in"=w9572) -> ("error out"=w9587:errorcluster, "Sync Box.lvclass"=w9588:refnum<class "Sync Box.lvclass">, "SPARC4_AC out"=w9576:refnum<class "S4GUI.lvclass">)  [unwired: 7 in]
        n4110 = call-dynamic "Read Trigger.lvclass.vi"("error in (no error)"=w9587, "Sync Box in"=w9588) -> ("error out"=w9585:errorcluster, "Trigger.lvclass"=w9586:refnum<class "Trigger.lvclass">, "Sync Box out"=w9579:refnum<class "Sync Box.lvclass">)  [unwired: 7 in]
        n4111 = call-dynamic "Read State Machine.vi"("error in (no error)"=w9585, "Device in"=w9586) -> ("error out"=w9583:errorcluster, "State Machine.lvclass"=w9584:refnum<class "State Machine.lvclass">, "Device out"=w9580:refnum<class "Trigger.lvclass">)  [unwired: 7 in]
        n4112 = call "Next State.vi"("error in (no error)"=w9583, "New_State"=u32 40, "State Machine in"=w9584) -> ("error out"=w9578:errorcluster, "State Machine out"=w9581:refnum<class "State Machine.lvclass">)  [unwired: 7 in]
        n4113 = call-dynamic "Write State Machine.vi"("error in (no error)"=w9578, "State Machine.lvclass"=w9581, "Device in"=w9580) -> ("error out"=w9574:errorcluster, "Device out"=w9573:refnum<class "Trigger.lvclass">)  [unwired: 7 in]
        n4114 = call-dynamic "Write Trigger.lvclass.vi"("error in (no error)"=w9574, "Trigger.lvclass"=w9573, "Sync Box in"=w9579) -> ("error out"=w9575:errorcluster, "Sync Box out"=w9577:refnum<class "Sync Box.lvclass">)  [unwired: 7 in]
        n4115 = call-dynamic "Write Sync Box.lvclass.vi"("error in (no error)"=w9575, "Sync Box.lvclass"=w9577, "SPARC4_AC in"=w9576) -> ("error out"=w9570:errorcluster, "SPARC4_AC out"=w9569:refnum<class "S4GUI.lvclass">)  [unwired: 7 in]
      }
      event "Select Trigger Mode": Value Change {
        n4116 = event-data() -> ("NewVal"=w9590:bool)  [unwired: 1 in, 2 out]
        n4117 = call-dynamic "Read Sync Box.lvclass.vi"("error in (no error)"=w9598, "SPARC4_AC in"=w9599) -> ("error out"=w9610:errorcluster, "Sync Box.lvclass"=w9611:refnum<class "Sync Box.lvclass">, "SPARC4_AC out"=w9603:refnum<class "S4GUI.lvclass">)  [unwired: 7 in]
        n4118 = call-dynamic "Read Trigger.lvclass.vi"("error in (no error)"=w9610, "Sync Box in"=w9611) -> ("error out"=w9591:errorcluster, "Trigger.lvclass"=w9594:refnum<class "Trigger.lvclass">, "Sync Box out"=w9606:refnum<class "Sync Box.lvclass">)  [unwired: 7 in]
        n4119 = call-dynamic "Write Trigger Mode Target.vi"("error in (no error)"=w9591, "Trigger Mode Target"=w9590, "Trigger in"=w9594) -> ("error out"=w9592:errorcluster, "Trigger out"=w9593:refnum<class "Trigger.lvclass">)  [unwired: 7 in]
        n4120 = call-dynamic "Read State Machine.vi"("error in (no error)"=w9592, "Device in"=w9593) -> ("error out"=w9595:errorcluster, "State Machine.lvclass"=w9596:refnum<class "State Machine.lvclass">, "Device out"=w9607:refnum<class "Trigger.lvclass">)  [unwired: 7 in]
        n4121 = call "Next State.vi"("error in (no error)"=w9595, "New_State"=u32 30, "State Machine in"=w9596) -> ("error out"=w9605:errorcluster, "State Machine out"=w9608:refnum<class "State Machine.lvclass">)  [unwired: 7 in]
        n4122 = call-dynamic "Write State Machine.vi"("error in (no error)"=w9605, "State Machine.lvclass"=w9608, "Device in"=w9607) -> ("error out"=w9601:errorcluster, "Device out"=w9600:refnum<class "Trigger.lvclass">)  [unwired: 7 in]
        n4123 = call-dynamic "Write Trigger.lvclass.vi"("error in (no error)"=w9601, "Trigger.lvclass"=w9600, "Sync Box in"=w9606) -> ("error out"=w9602:errorcluster, "Sync Box out"=w9604:refnum<class "Sync Box.lvclass">)  [unwired: 7 in]
        n4124 = call-dynamic "Write Sync Box.lvclass.vi"("error in (no error)"=w9602, "Sync Box.lvclass"=w9604, "SPARC4_AC in"=w9603) -> ("error out"=w9597:errorcluster, "SPARC4_AC out"=w9589:refnum<class "S4GUI.lvclass">)  [unwired: 7 in]
      }
      event "Set SyncBox": Value Change {
        n4125 = event-data() -> ()  [unwired: 1 in, 4 out]
        n4126 = call-dynamic "Read Sync Box.lvclass.vi"("error in (no error)"=w9614, "SPARC4_AC in"=w9615) -> ("error out"=w9630:errorcluster, "Sync Box.lvclass"=w9631:refnum<class "Sync Box.lvclass">, "SPARC4_AC out"=w9619:refnum<class "S4GUI.lvclass">)  [unwired: 7 in]
        n4127 = call-dynamic "Read Trigger.lvclass.vi"("error in (no error)"=w9630, "Sync Box in"=w9631) -> ("error out"=w9628:errorcluster, "Trigger.lvclass"=w9629:refnum<class "Trigger.lvclass">, "Sync Box out"=w9622:refnum<class "Sync Box.lvclass">)  [unwired: 7 in]
        n4128 = call-dynamic "Read State Machine.vi"("error in (no error)"=w9628, "Device in"=w9629) -> ("error out"=w9626:errorcluster, "State Machine.lvclass"=w9627:refnum<class "State Machine.lvclass">, "Device out"=w9623:refnum<class "Trigger.lvclass">)  [unwired: 7 in]
        n4129 = call "Next State.vi"("error in (no error)"=w9626, "New_State"=u32 10, "State Machine in"=w9627) -> ("error out"=w9621:errorcluster, "State Machine out"=w9624:refnum<class "State Machine.lvclass">)  [unwired: 7 in]
        n4130 = call-dynamic "Write State Machine.vi"("error in (no error)"=w9621, "State Machine.lvclass"=w9624, "Device in"=w9623) -> ("error out"=w9617:errorcluster, "Device out"=w9616:refnum<class "Trigger.lvclass">)  [unwired: 7 in]
        n4131 = call-dynamic "Write Trigger.lvclass.vi"("error in (no error)"=w9617, "Trigger.lvclass"=w9616, "Sync Box in"=w9622) -> ("error out"=w9618:errorcluster, "Sync Box out"=w9620:refnum<class "Sync Box.lvclass">)  [unwired: 7 in]
        n4132 = call-dynamic "Write Sync Box.lvclass.vi"("error in (no error)"=w9618, "Sync Box.lvclass"=w9620, "SPARC4_AC in"=w9619) -> ("error out"=w9613:errorcluster, "SPARC4_AC out"=w9612:refnum<class "S4GUI.lvclass">)  [unwired: 7 in]
      }
      event "Set Focus": Value Change {
        n4133 = event-data() -> ("NewVal"=w9632:bool)  [unwired: 1 in]
        n4134 = case shown="True" w9632 {
          tunnel: w9636 -> [w9638 w9647]
          tunnel: w9635 -> [w9637 w9646]
          tunnel: [w9637 w9645] -> w9634
          tunnel: [w9638 w9644] -> w9633
          frame False {
          }
          frame True {
            n4135 = call-dynamic "Read TelFocus.lvclass.vi"("error in (no error)"=w9646, "S4GUI in"=w9647) -> ("error out"=w9660:errorcluster, "TelFocus.lvclass"=w9661:refnum<class "TelFocus.lvclass">, "S4GUI out"=w9651:refnum<class "S4GUI.lvclass">)  [unwired: 7 in]
            n4136 = call-dynamic "Read SecMirror.lvclass.vi"("error in (no error)"=w9660, "TelFocus in"=w9661) -> ("error out"=w9640:errorcluster, "SecMirror.lvclass"=w9643:refnum<class "SecMirror.lvclass">, "TelFocus out"=w9654:refnum<class "TelFocus.lvclass">)  [unwired: 7 in]
            n4137 = call-dynamic "Write target.vi"("error in (no error)"=w9640, "target"="Target focus", "SecMirror in"=w9643) -> ("error out"=w9639:errorcluster, "SecMirror out"=w9642:refnum<class "SecMirror.lvclass">)  [unwired: 7 in]
            n4138 = call-dynamic "Read State Machine.vi"("error in (no error)"=w9639, "Device in"=w9642) -> ("error out"=w9658:errorcluster, "State Machine.lvclass"=w9659:refnum<class "State Machine.lvclass">, "Device out"=w9655:refnum<class "SecMirror.lvclass">)  [unwired: 7 in]
            n4139 = call "Next State.vi"("error in (no error)"=w9658, "New_State"=1, "State Machine in"=w9659) -> ("error out"=w9653:errorcluster, "State Machine out"=w9656:refnum<class "State Machine.lvclass">)  [unwired: 7 in]
            n4140 = call-dynamic "Write State Machine.vi"("error in (no error)"=w9653, "State Machine.lvclass"=w9656, "Device in"=w9655) -> ("error out"=w9649:errorcluster, "Device out"=w9648:refnum<class "SecMirror.lvclass">)  [unwired: 7 in]
            n4141 = call-dynamic "Write SecMirror.lvclass.vi"("error in (no error)"=w9649, "SecMirror.lvclass"=w9648, "TelFocus in"=w9654) -> ("error out"=w9650:errorcluster, "TelFocus out"=w9652:refnum<class "TelFocus.lvclass">)  [unwired: 7 in]
            n4142 = call-dynamic "Write TelFocus.lvclass.vi"("error in (no error)"=w9650, "TelFocus.lvclass"=w9652, "S4GUI in"=w9651) -> ("error out"=w9645:errorcluster, "S4GUI out"=w9644:refnum<class "S4GUI.lvclass">)  [unwired: 7 in]
          }
        }
      }
      event "Set Focus 2": Value Change {
        n4143 = event-data() -> ("NewVal"=w9662:bool)  [unwired: 1 in]
        n4144 = case shown="True" w9662 {
          tunnel: w9666 -> [w9668 w9677]
          tunnel: w9665 -> [w9667 w9676]
          tunnel: [w9667 w9675] -> w9664
          tunnel: [w9668 w9674] -> w9663
          frame False {
          }
          frame True {
            n4145 = call-dynamic "Read TelFocus.lvclass.vi"("error in (no error)"=w9676, "S4GUI in"=w9677) -> ("error out"=w9690:errorcluster, "TelFocus.lvclass"=w9691:refnum<class "TelFocus.lvclass">, "S4GUI out"=w9681:refnum<class "S4GUI.lvclass">)  [unwired: 7 in]
            n4146 = call-dynamic "Read SecMirror.lvclass.vi"("error in (no error)"=w9690, "TelFocus in"=w9691) -> ("error out"=w9671:errorcluster, "SecMirror.lvclass"=w9673:refnum<class "SecMirror.lvclass">, "TelFocus out"=w9684:refnum<class "TelFocus.lvclass">)  [unwired: 7 in]
            n4147 = call-dynamic "Write target.vi"("error in (no error)"=w9671, "target"="Target focus 2", "SecMirror in"=w9673) -> ("error out"=w9670:errorcluster, "SecMirror out"=w9672:refnum<class "SecMirror.lvclass">)  [unwired: 7 in]
            n4148 = call-dynamic "Read State Machine.vi"("error in (no error)"=w9670, "Device in"=w9672) -> ("error out"=w9688:errorcluster, "State Machine.lvclass"=w9689:refnum<class "State Machine.lvclass">, "Device out"=w9685:refnum<class "SecMirror.lvclass">)  [unwired: 7 in]
            n4149 = call "Next State.vi"("error in (no error)"=w9688, "New_State"=1, "State Machine in"=w9689) -> ("error out"=w9683:errorcluster, "State Machine out"=w9686:refnum<class "State Machine.lvclass">)  [unwired: 7 in]
            n4150 = call-dynamic "Write State Machine.vi"("error in (no error)"=w9683, "State Machine.lvclass"=w9686, "Device in"=w9685) -> ("error out"=w9679:errorcluster, "Device out"=w9678:refnum<class "SecMirror.lvclass">)  [unwired: 7 in]
            n4151 = call-dynamic "Write SecMirror.lvclass.vi"("error in (no error)"=w9679, "SecMirror.lvclass"=w9678, "TelFocus in"=w9684) -> ("error out"=w9680:errorcluster, "TelFocus out"=w9682:refnum<class "TelFocus.lvclass">)  [unwired: 7 in]
            n4152 = call-dynamic "Write TelFocus.lvclass.vi"("error in (no error)"=w9680, "TelFocus.lvclass"=w9682, "S4GUI in"=w9681) -> ("error out"=w9675:errorcluster, "S4GUI out"=w9674:refnum<class "S4GUI.lvclass">)  [unwired: 7 in]
          }
        }
      }
      event "Stop Focus", "Stop Focus 2": Value Change {
        n4153 = event-data() -> ("NewVal"=w9692:bool)  [unwired: 1 in]
        n4154 = case shown="True" w9692 {
          tunnel: w9696 -> [w9698 w9704]
          tunnel: w9695 -> [w9697 w9703]
          tunnel: [w9697 w9702] -> w9694
          tunnel: [w9698 w9701] -> w9693
          frame False {
          }
          frame True {
            n4155 = call-dynamic "Read TelFocus.lvclass.vi"("error in (no error)"=w9703, "S4GUI in"=w9704) -> ("error out"=w9717:errorcluster, "TelFocus.lvclass"=w9718:refnum<class "TelFocus.lvclass">, "S4GUI out"=w9708:refnum<class "S4GUI.lvclass">)  [unwired: 7 in]
            n4156 = call-dynamic "Read SecMirror.lvclass.vi"("error in (no error)"=w9717, "TelFocus in"=w9718) -> ("error out"=w9699:errorcluster, "SecMirror.lvclass"=w9700:refnum<class "SecMirror.lvclass">, "TelFocus out"=w9711:refnum<class "TelFocus.lvclass">)  [unwired: 7 in]
            n4157 = call-dynamic "Read State Machine.vi"("error in (no error)"=w9699, "Device in"=w9700) -> ("error out"=w9715:errorcluster, "State Machine.lvclass"=w9716:refnum<class "State Machine.lvclass">, "Device out"=w9712:refnum<class "SecMirror.lvclass">)  [unwired: 7 in]
            n4158 = call "Next State.vi"("error in (no error)"=w9715, "New_State"=10, "State Machine in"=w9716) -> ("error out"=w9710:errorcluster, "State Machine out"=w9713:refnum<class "State Machine.lvclass">)  [unwired: 7 in]
            n4159 = call-dynamic "Write State Machine.vi"("error in (no error)"=w9710, "State Machine.lvclass"=w9713, "Device in"=w9712) -> ("error out"=w9706:errorcluster, "Device out"=w9705:refnum<class "SecMirror.lvclass">)  [unwired: 7 in]
            n4160 = call-dynamic "Write SecMirror.lvclass.vi"("error in (no error)"=w9706, "SecMirror.lvclass"=w9705, "TelFocus in"=w9711) -> ("error out"=w9707:errorcluster, "TelFocus out"=w9709:refnum<class "TelFocus.lvclass">)  [unwired: 7 in]
            n4161 = call-dynamic "Write TelFocus.lvclass.vi"("error in (no error)"=w9707, "TelFocus.lvclass"=w9709, "S4GUI in"=w9708) -> ("error out"=w9702:errorcluster, "S4GUI out"=w9701:refnum<class "S4GUI.lvclass">)  [unwired: 7 in]
          }
        }
      }
      event "cooler ON 1": Value Change {
        n4162 = event-data() -> ("NewVal"=w9719:bool)  [unwired: 1 in]
        n4163 = case shown="True" w9719 {
          tunnel: [w9724 w9759] -> w9723
          tunnel: [w9725 w9758] -> w9722
          tunnel: w9721 -> [w9725 w9729]
          tunnel: w9720 -> [w9724 w9728]
          frame False {
          }
          frame True {
            w9727 = i16 1 items=["Cooler OFF", "Cooler ON"] ("Cooler ON/OFF")
            n4164 = Concatenate Strings("SET COOLER " ("User Event"), "ON ", "CLICKED - CH1" ("User Event")) -> (w9731:string)
            n4165 = call-dynamic "Write User Event.vi"("error in (no error)"=w9728, "User Event"=w9731, "S4GUI in"=w9729) -> ("error out"=w9732:errorcluster, "S4GUI out"=w9734:refnum<class "S4GUI.lvclass">)  [unwired: 7 in]
            n4166 = call-dynamic "Read AcquisitionA.vi"("error in (no error)"=w9732, "S4ACS_GUI in"=w9734) -> ("error out"=w9756:errorcluster, "Acquisition.lvclass"=w9757:refnum<class "Acquisition.lvclass">, "S4ACS_GUI out"=w9747:refnum<class "S4GUI.lvclass">)  [unwired: 7 in]
            n4167 = call-dynamic "Read Channel.vi"("error in (no error)"=w9756, "Acquisition in"=w9757) -> ("error out"=w9740:errorcluster, "Channel.lvclass"=w9744:refnum<class "Channel.lvclass">, "Acquisition out"=w9750:refnum<class "Acquisition.lvclass">)  [unwired: 7 in]
            n4168 = call-dynamic "Read Interface.vi"("error in (no error)"=w9740, "Channel in"=w9744) -> ("error out"=w9735:errorcluster, "Interface.lvclass"=w9736:refnum<class "Interface.lvclass">, "Channel out"=w9743:refnum<class "Channel.lvclass">)  [unwired: 7 in]
